vi "FB Switch Input Error.vi"(8 "error in":errorcluster) -> (0 "error out":errorcluster)   [LabVIEW 2020]
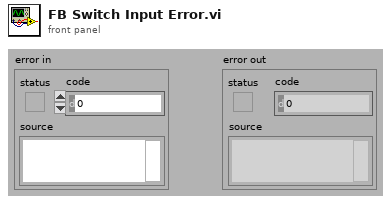
[diagram p1: front panel]
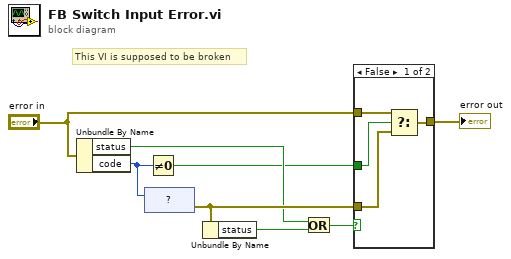
[diagram p0: block diagram]
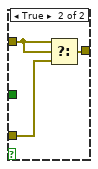
[diagram p2: hidden frame]
diagram:
  # "This VI is supposed to be broken"
  n1 = Unbundle By Name("error in") -> ("status"=w6:bool, "code"=w2:i32)
  n2 = shared-variable "?"(w2) -> (error out=w7:errorcluster)  [unwired: 1 in]
  n3 = Not Equal To 0?(x=w2) -> (x != 0?=w3:bool)
  n4 = Unbundle By Name(w7) -> ("status"=w5:bool)
  n5 = Or(x=w6, y=w5) -> (x .or. y?=w4:bool)
  n6 = case shown="False" w4 {
    tunnel: "error in" -> [w12 w13]
    tunnel: [w9 w15] -> w1
    tunnel: w7 -> [w10 w14]
    tunnel: w3 -> [w11 _]
    frame False {
      n7 = Select(t=w12, s=w11, f=w10) -> (s? t:f=w9:errorcluster)
    }
    frame True {
      n8 = Select(t=w13, s=w13, f=w14) -> (s? t:f=w15:errorcluster)
    }
  }
  "error out" <- w1
